vi "Connect.vi"(6 "wait for reply (T)":bool=TRUE, 8 "error in":errorcluster, 9 "COM params":T1={"baud rate"=9600, "data bits"=8, "parity"=enum."None", "stop bits"=10, "flow control"=0} {"stop bits" items=["1.0"=10, "1.5"=15, "2.0"=20]; "flow control" items=["None", "XON/XOFF", "RTS/CTS", "XON/XOFF & RTS/CTS", "DTR/DSR", "XON/XOFF & DTR/DSR"]}, 10 "VISA resource":refnum<visa-resource-name>, 11 "Module ID":i32=-1) -> (0 "error out":errorcluster, 1 "timed out?":bool)   [LabVIEW 2020, in "Arduino stepper.lvlib"]
doc: "Request to connect to Arduino device using given communication parameters.\n_____\nCreated using DQMH Event Scripter 6.1.0.128."
uses:
  Arduino stepper.lvlib
  Support/COM params--typedef.ctl
  Connect Argument--cluster.ctl
  Connect (Reply Payload)--cluster.ctl
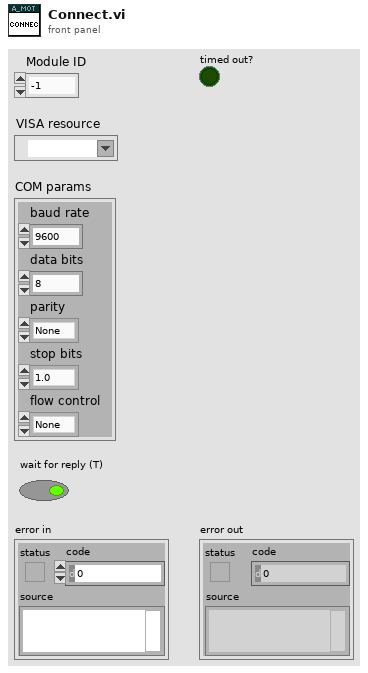
[diagram p1: front panel]
types:
  T1 = typedef "Arduino stepper.lvlib/COM params--typedef.ctl" = cluster{"baud rate":u32, "data bits":u16, "parity":enum16{"None", "Odd", "Even", "Mark", "Space"}, "stop bits":u16, "flow control":u16}
  T2 = typedef "Arduino stepper.lvlib/Connect Argument--cluster.ctl" = cluster{"Module ID":i32, "VISA resource":refnum<visa-resource-name>, "COM params":T1, "Wait Notifier":refnum<notifier>, "wait for reply":bool}
  T3 = typedef "Arduino stepper.lvlib/Request Events--cluster.ctl" = cluster{"Stop Module":refnum<user-event>, "Show Panel":refnum<user-event>, "Hide Panel":refnum<user-event>, "Show Diagram":refnum<user-event>, "Get Module Execution Status":refnum<user-event>, "Connect":refnum<user-event>, "Disconnect":refnum<user-event>, "Move motor":refnum<user-event>, "Get position":refnum<user-event>, "Read port continuously":refnum<user-event>, "Stop continuous reading":refnum<user-event>, "Stop motor":refnum<user-event>, "Read end-stops":refnum<user-event>, "Read all info":refnum<user-event>}
  T4 = typedef "Arduino stepper.lvlib/Connect (Reply Payload)--cluster.ctl" = cluster{"error":errorcluster}
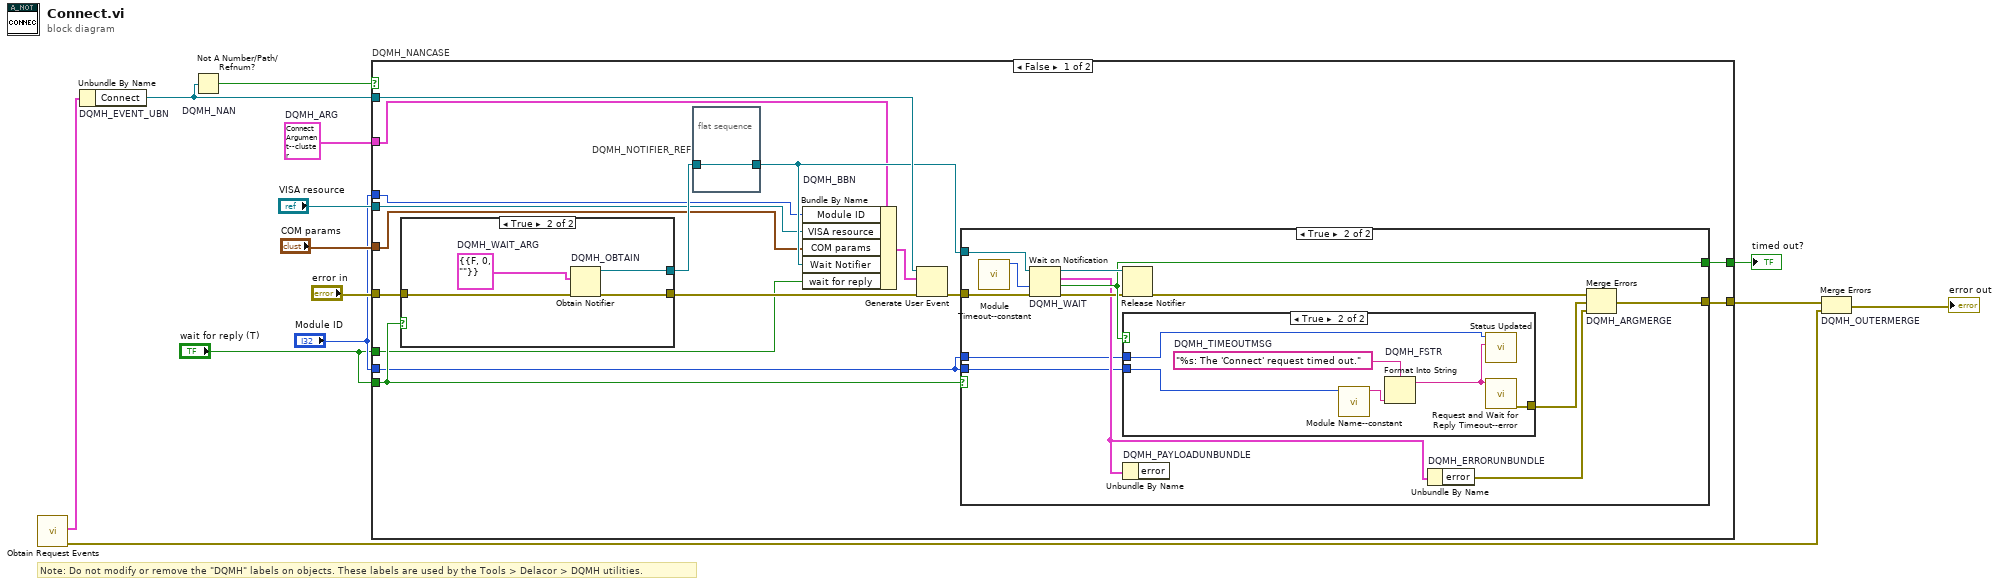
[diagram p0: block diagram]
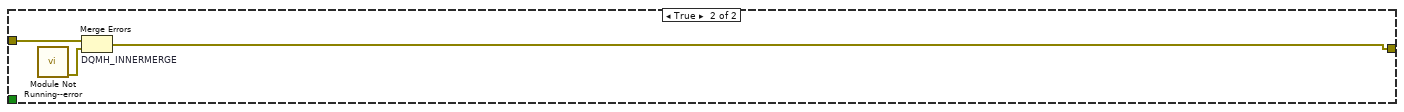
[diagram p5: hidden frame]
diagram:
  w7 = T2 {"Module ID"=-1, "VISA resource"="", "COM params"={"baud rate"=9600, "data bits"=8, "parity"=enum."None", "stop bits"=10, "flow control"=0}, "Wait Notifier"=refnum, "wait for reply"=FALSE}  # DQMH_ARG
  # "Note: Do not modify or remove the \"DQMH\" labels on objects. These labels are used by the Tools > Delacor > DQMH utilities."
  n1 = call "Obtain Request Events.vi"() -> ("error out"=w2:errorcluster, "Arduino stepper Request Events"=w1:T3)  [unwired: 10 in]
  n2 = Unbundle By Name "DQMH_EVENT_UBN"(w1) -> ("Connect"=w8:refnum<user-event>)
  n3 = Not A Number/Path/Refnum? "DQMH_NAN"(number/path/refnum=w8) -> (NaN/Path/Refnum?=w9:bool)
  n4 = case "DQMH_NANCASE" shown="False" w9 {
    tunnel: "error in" -> [w29 w58]
    tunnel: w8 -> [w27 _]
    tunnel: [w24 w57] -> w10
    tunnel: [w25 _] -> w12
    tunnel: "wait for reply (T)" -> [w22 _]
    tunnel: w7 -> [w19 _]
    tunnel: "Module ID" -> [w18 _]
    tunnel: "VISA resource" -> [w17 _]
    tunnel: "COM params" -> [w16 _]
    tunnel: "Module ID" -> [w15 _]
    tunnel: "wait for reply (T)" -> [w14 _]
    frame False {
      n5 = case shown="True" w22 {
        tunnel: w29 -> [w51 w55]
        tunnel: [w51 w54] -> w26
        tunnel: [_ w52] -> w21
        frame False {
        }
        frame True {
          w53 = T4 {"error"={"status"=FALSE, "code"=0, "source"=""}}  # DQMH_WAIT_ARG
          n6 = Obtain Notifier "DQMH_OBTAIN"(notification data type=w53, error in (no error)=w55) -> (notifier out=w52:refnum<notifier>, error out=w54:errorcluster)  [unwired: 2 in, 1 out]
        }
      }
      n7 = flat-sequence "DQMH_NOTIFIER_REF" {
        tunnel: w21 -> [w30]
        tunnel: [w30] -> w20
        frame #0 {
        }
      }
      n8 = Bundle By Name "DQMH_BBN"(cluster=w19, "Module ID"=w18, "VISA resource"=w17, "COM params"=w16, "Wait Notifier"=w20, "wait for reply"=w14) -> (w23:T2)
      n9 = Generate User Event(user event=w27, event data cluster=w23, error in=w26) -> (error out=w28:errorcluster)  [unwired: 1 in, 1 out]
      n10 = case shown="True" w22 {
        tunnel: w28 -> [w31 w44]
        tunnel: w20 -> [_ w43]
        tunnel: [_ w41] -> w25
        tunnel: [w31 w40] -> w24
        tunnel: w15 -> [_ w33]
        tunnel: w15 -> [_ w32]
        frame False {
        }
        frame True {
          n11 = call "Module Timeout--constant.vi"() -> ("Module Timeout"=w34:i32)  [unwired: 11 in]
          n12 = Wait on Notification "DQMH_WAIT"(notifier=w43, timeout in ms (-1)=w34, error in (no error)=w44) -> (notifier out=w42:refnum<notifier>, notification=w35:T4, timed out?=w41:bool, error out=w39:errorcluster)  [unwired: 1 in]
          n13 = Release Notifier(notifier=w42, error in (no error)=w39) -> (error out=w38:errorcluster)  [unwired: 1 in, 2 out]
          n14 = case shown="True" w41 {
            tunnel: [_ w48] -> w36
            tunnel: w33 -> [_ w46]
            tunnel: w32 -> [_ w45]
            frame False {
            }
            frame True {
              w50 = "%s: The 'Connect' request timed out."  # DQMH_TIMEOUTMSG
              n15 = call "Module Name--constant.vi"("Module ID"=w45) -> ("Module Name"=w47:string)  [unwired: 10 in]
              n16 = Format Into String "DQMH_FSTR"(format string=w50, w47) -> (resulting string=w49:string)  [unwired: 2 in, 1 out]
              n17 = call "Status Updated.vi"("Status"=w49, "Module ID"=w46) -> ()  [unwired: 9 in, 1 out]
              n18 = call "Request and Wait for Reply Timeout--error.vi"("Error Message"=w49) -> ("error out"=w48:errorcluster)  [unwired: 10 in]
            }
          }
          n19 = Unbundle By Name "DQMH_PAYLOADUNBUNDLE"(w35) -> ()  [unwired: 1 out]
          n20 = Unbundle By Name "DQMH_ERRORUNBUNDLE"(w35) -> ("error"=w37:errorcluster)
          n21 = Merge Errors "DQMH_ARGMERGE"(w38, w36, w37) -> (w40:errorcluster)
        }
      }
    }
    frame True {
      n22 = call "Module Not Running--error.vi"() -> ("error out"=w56:errorcluster)  [unwired: 11 in]
      n23 = Merge Errors "DQMH_INNERMERGE"(w58, w56) -> (w57:errorcluster)
    }
  }
  "timed out?" <- w12
  n24 = Merge Errors "DQMH_OUTERMERGE"(w10, w2) -> (→"error out":errorcluster)
